vi "GetRoom.vi"(7 "LabVIEW Web Service Request":refnum<class "Web Request.lvclass">, 9 "Command":string, 10 "Room":i32) -> (2 "Response":string)   [LabVIEW 2015]
uses:
  <vilib>/wsapi/Web Request.lvclass
  LVRestAPI/TypeDef/GetRoomCommands.ctl
  TypeDef/RoomsActionEnum.ctl
  LVRestAPI/RestApi.lvlib
panel:
  out "postdata":string
  # "Use the Web Service Request input terminal to call the VIs on the Web Services palette. Do not remove it from the connector pane unless you don't need access to the palette."
  # "Each additional control wired to the connector pane will be available as an input in the URL. To include an indicator in terminal-mode output (the default setting), it must also be wired to the connector pane."
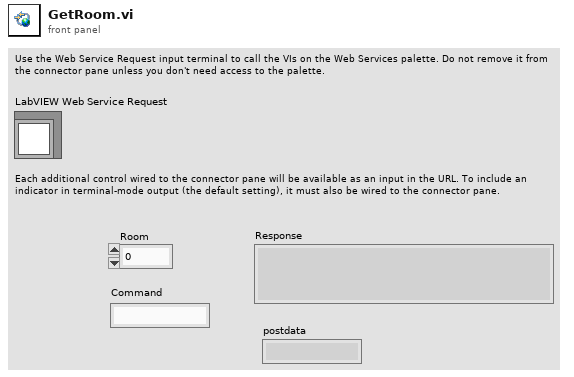
[diagram p1: front panel]
types:
  T1 = typedef "RestApi.lvlib/GetRoomCommands.ctl" = enum16{"ReadRoom", "ReadFlag", "ReadFlagState", "ReadFlagColor", "ReadBedVacant", "ReadPersonnel", "ReadRequests", "ReadBeaconID", "ReadBedURL", "ReadRoomsNumbers"}
  T2 = typedef "RoomsActionEnum.ctl" = enum16{"Init", "Add Room", "Remove Room", "Read Room", "Read Flag", "Read Flag State", "Write Flag State", "Read Flag Color", "Write Flag Color", "Read Bed Vacant", "Write Bed Vacant", "Read Personnel", "Add Personnel", "Remove Personnel", "Read Requests", "Add Request", "Remove Request", "Read Beacon ID", "Write Beacon ID", "Write Bed URL", "Read Bed URL", "Read Rooms Numbers"}
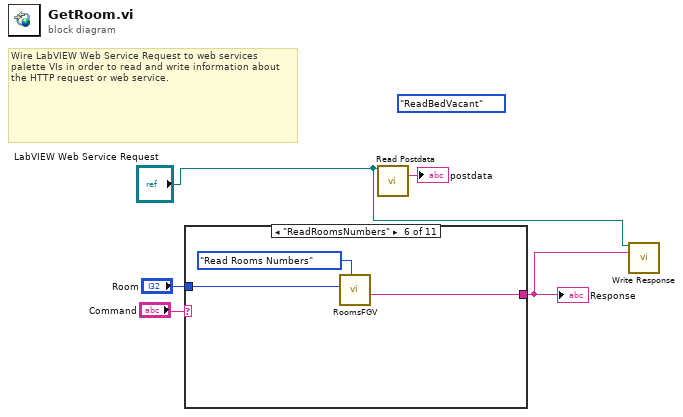
[diagram p0: block diagram]
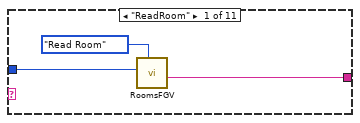
[diagram p2: hidden frame]
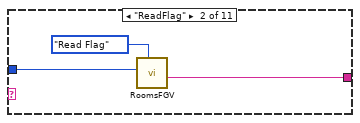
[diagram p3: hidden frame]
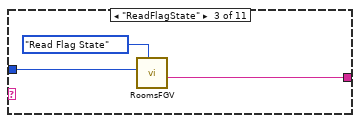
[diagram p4: hidden frame]
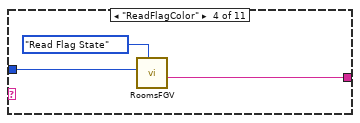
[diagram p5: hidden frame]
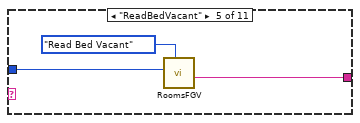
[diagram p6: hidden frame]
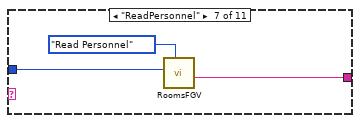
[diagram p7: hidden frame]
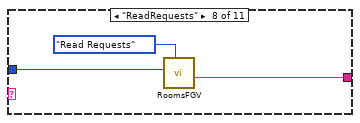
[diagram p8: hidden frame]
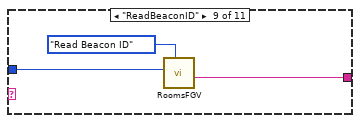
[diagram p9: hidden frame]
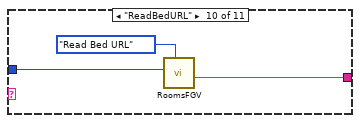
[diagram p10: hidden frame]
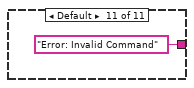
[diagram p11: hidden frame]
diagram:
  (unwired) GetRoomCommands."ReadBedVacant" ("Room Commands")
  # "Wire LabVIEW Web Service Request to web services palette VIs in order to read and write information about the HTTP request or web service."
  n1 = case shown="\"ReadRoomsNumbers\"" "Command" {
    tunnel: "Room" -> [w7 w10 w13 w16 w19 w23 w25 w28 w31 w34 _]
    tunnel: [w6 w9 w12 w15 w18 w22 w24 w27 w30 w33 "Error: Invalid Command" ("Data Out")] -> w2
    frame "ReadRoom" {
      n2 = call "RoomsFGV.vi"("Actions"=RoomsActionEnum."Read Room", "Room"=w7) -> ("Data Out"=w6:string)  [unwired: 8 in, 1 out]
    }
    frame "ReadFlag" {
      n3 = call "RoomsFGV.vi"("Actions"=RoomsActionEnum."Read Flag", "Room"=w10) -> ("Data Out"=w9:string)  [unwired: 8 in, 1 out]
    }
    frame "ReadFlagState" {
      n4 = call "RoomsFGV.vi"("Actions"=RoomsActionEnum."Read Flag State", "Room"=w13) -> ("Data Out"=w12:string)  [unwired: 8 in, 1 out]
    }
    frame "ReadFlagColor" {
      n5 = call "RoomsFGV.vi"("Actions"=RoomsActionEnum."Read Flag State", "Room"=w16) -> ("Data Out"=w15:string)  [unwired: 8 in, 1 out]
    }
    frame "ReadBedVacant" {
      n6 = call "RoomsFGV.vi"("Actions"=RoomsActionEnum."Read Bed Vacant", "Room"=w19) -> ("Data Out"=w18:string)  [unwired: 8 in, 1 out]
    }
    frame "ReadRoomsNumbers" {
      n7 = call "RoomsFGV.vi"("Actions"=RoomsActionEnum."Read Rooms Numbers", "Room"=w23) -> ("Data Out"=w22:string)  [unwired: 8 in, 1 out]
    }
    frame "ReadPersonnel" {
      n8 = call "RoomsFGV.vi"("Actions"=RoomsActionEnum."Read Personnel", "Room"=w25) -> ("Data Out"=w24:string)  [unwired: 8 in, 1 out]
    }
    frame "ReadRequests" {
      n9 = call "RoomsFGV.vi"("Actions"=RoomsActionEnum."Read Requests", "Room"=w28) -> ("Data Out"=w27:string)  [unwired: 8 in, 1 out]
    }
    frame "ReadBeaconID" {
      n10 = call "RoomsFGV.vi"("Actions"=RoomsActionEnum."Read Beacon ID", "Room"=w31) -> ("Data Out"=w30:string)  [unwired: 8 in, 1 out]
    }
    frame "ReadBedURL" {
      n11 = call "RoomsFGV.vi"("Actions"=RoomsActionEnum."Read Bed URL", "Room"=w34) -> ("Data Out"=w33:string)  [unwired: 8 in, 1 out]
    }
    frame Default {
    }
  }
  "Response" <- w2
  n12 = call <vilib>:"Read Postdata.vi"("LabVIEW Web Service Request"="LabVIEW Web Service Request") -> ("postdata"=→"postdata":string)  [unwired: 12 in, 2 out]
  n13 = call <vilib>:"Write Response.vi"("LabVIEW Web Service Request"="LabVIEW Web Service Request", "response string"=w2) -> ()  [unwired: 12 in, 2 out]
